vi "realtime_fault_detect.vi"(1 "control":bool, 2 "enable":bool, 3 "timeout":u32=5) -> (0 "timeout":bool)   [LabVIEW 2018]
uses:
  <vilib>/rvi/eio/common/nirviEmuTemplateMethod_errors.vi
  <vilib>/eio/EIONode/EIONode.xnode
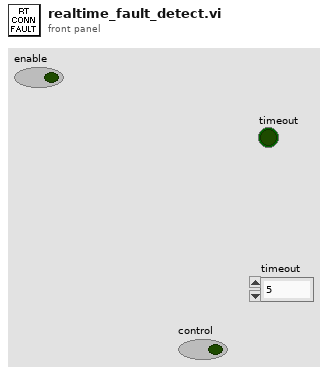
[diagram p1: front panel]
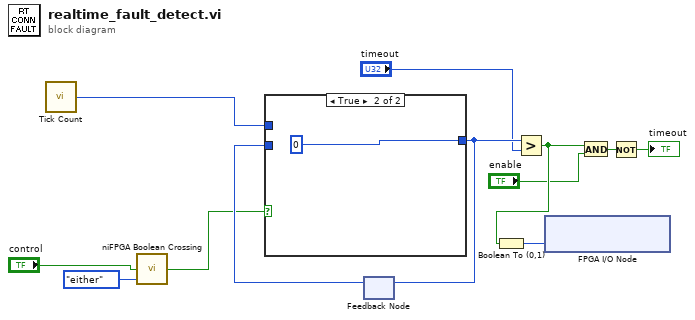
[diagram p0: block diagram]
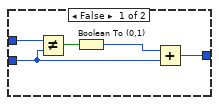
[diagram p2: hidden frame]
diagram:
  n1 = call "Tick Count"() -> ("Tick Count(mSec)"=w10:u8)
  n2 = call <vilib>:"niFPGA Boolean Crossing.vi"("input"="control", "direction"=enum8{"either", "false-true", "true-false"}."either") -> ("crossing"=w5:bool)  [unwired: 7 in]
  n3 = feedback #1() -> (w11:u8)  [unwired: 1 in]
  n4 = case shown="True" w5 {
    tunnel: w11 -> [w14 _]
    tunnel: [w13 u8 0 ("Numeric")] -> w9
    tunnel: w10 -> [w15 _]
    frame False {
      n5 = Not Equal?(x=w15, y=w14) -> (x != y?=w17:bool)
      n6 = Boolean To (0,1)(Boolean=w17) -> (0, 1=w16:i16)
      n7 = Add(x=w16, y=w14) -> (x+y=w13:i16)
    }
    frame True {
    }
  }
  n8 = feedback-in #1(w9) -> ()
  n9 = Greater?(x=w9, y="timeout") -> (0:w4:bool)
  n10 = Boolean To (0,1)(Boolean=w4) -> (0, 1=w7:i16)
  n11 = xnode "FPGA I/O Node"("USER FPGA LED"=w7) -> ()  [unwired: 1 in, 1 out]
  n12 = And(x=w4, y="enable") -> (x .and. y?=w2:bool)
  n13 = Not(x=w2) -> (.not. x?=→"timeout":bool)
